vi "Image Processing with Vision Assistant (FPGA)-useFIFO1out.vi"() -> ()   [LabVIEW 2016]
uses:
  <vilib>/visionFPGA/Controls/IMAQ FPGA Image Size.ctl
  <vilib>/rvi/Emulation/niFpgaSctlEmulationGetInTimedLoop.vi
  <vilib>/rvi/Emulation/niFpgaProcessEmulError.vi
  <vilib>/rvi/Emulation/niFpgaGetClockAttributes.vi
  <vilib>/rvi/Emulation/niFpgaEmulationReportErrorSimple.vi
  <vilib>/rvi/eio/common/nirviEmuTemplateMethod_errors.vi
  <vilib>/rvi/interface/RandomDataEmulation/niFpgaRandomDataHandleErrors.vi
  <vilib>/rvi/DataTransferAndStorage/Container/Common/niFpgaContainerGetUniqueNameForEmu.vi
  <vilib>/rvi/DataTransferAndStorage/Container/Common/niFpgaContainerSetEmuInfo.vi
  <vilib>/rvi/eio/common/nirviEmuReportErrorAndStop.vi
  <vilib>/rvi/DataTransferAndStorage/Container/Common/niFpgaContainerExecOnDevCompGetState.vi
  <vilib>/rvi/Emulation/niFpgaEmulationIsFPGAContextNoSignature.vi
  <vilib>/rvi/errors/niFpgaSetErrorForExecOnDevCompSimple.vi
  <vilib>/rvi/FIFO/Fifo_Resource/nirvififoEmulationSetSize.vi
  <vilib>/rvi/FIFO/Fifo_Resource/nirviFifoEmulationQueueMgr.vi
  <instcachedir>/0/nirviFifoEmulationQueueMgr_E5CAEC123FF24DC58D834DCA3CDAA9B5.lvgen/nirviFifoEmulationQueueMgr_E5CAEC123FF24DC58D834DCA3CDAA9B5_002.vi
  <vilib>/rvi/FIFO/Fifo_Resource/nirvififoEmulationDetermineInputValidOut.vi
  <vilib>/rvi/FIFO/Fifo_Resource/nirvififoEmulationCreateLock.vi
  <vilib>/rvi/FIFO/Fifo_Resource/nirvififoEmulationObtainLock.vi
  <vilib>/rvi/FIFO/Fifo_Resource/nirvififoEmulationReleaseLock.vi
  <vilib>/rvi/occurrence/nirviWaitOnOccurrenceBase.vi
  <vilib>/rvi/errors/nirviReportUnexpectedCaseInternalError.vi
  <vilib>/rvi/errors/nirviReportUnexpectedCaseInternalError (U32).vi
  <vilib>/Utility/error.llb/Clear Errors.vi
  <vilib>/rvi/Emulation/niFpgaCriticalErrorInLSC.vi
  <vilib>/eio/EIONode/EIONode.xnode
  <vilib>/rvi/DataTransferAndStorage/Container/XNode/niFpgaContainer.xnode
  <vilib>/rvi/interface/RandomDataEmulation/nirviRandomDataFpgaReadWriteTemplate.vi
  <vilib>/rvi/LocalResourceManager/LocalResourceManager.xnode
  <vilib>/rvi/FIFO/Fifo_Resource/niFpgaFifoEmulationRefIn.vi
panel:
  out "OutputType":u8
  out "CanSendImage":bool=TRUE
  out "Mode LED Status":bool=TRUE
  out "Radio LED Status":bool=TRUE
  out "outputExtreme2":bool=TRUE
  out "outputExtreme1":bool=TRUE
  out "outputDOG2":bool=TRUE
  out "outputDOG1":bool=TRUE
  out "Ready For Output":bool=TRUE
  out "StartOfImage":bool=TRUE
  in  "Image Size":T1={"Width"=640, "Height"=480}
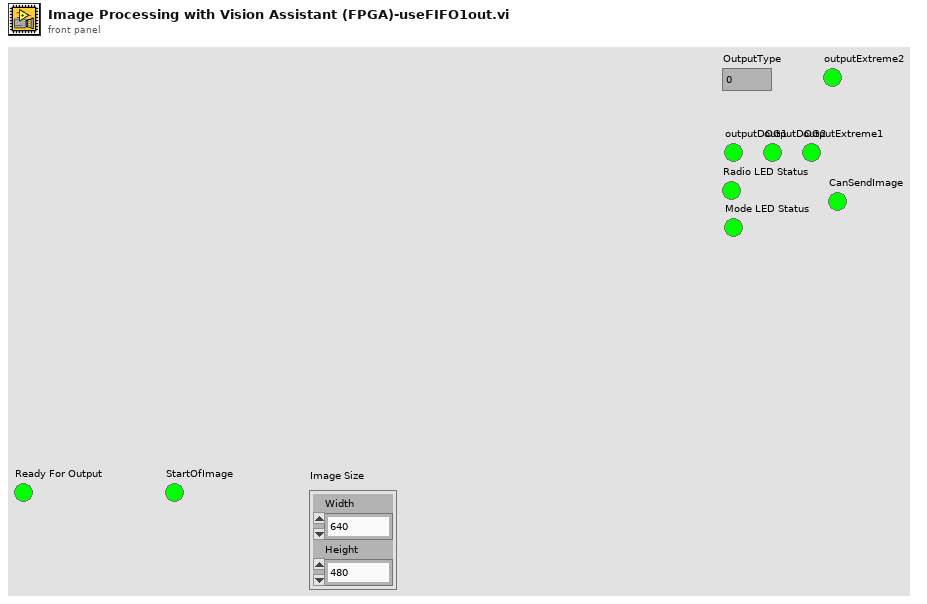
[diagram p1: front panel]
types:
  T1 = typedef "IMAQ FPGA Image Size.ctl" = cluster{"Width":u32, "Height":u32}
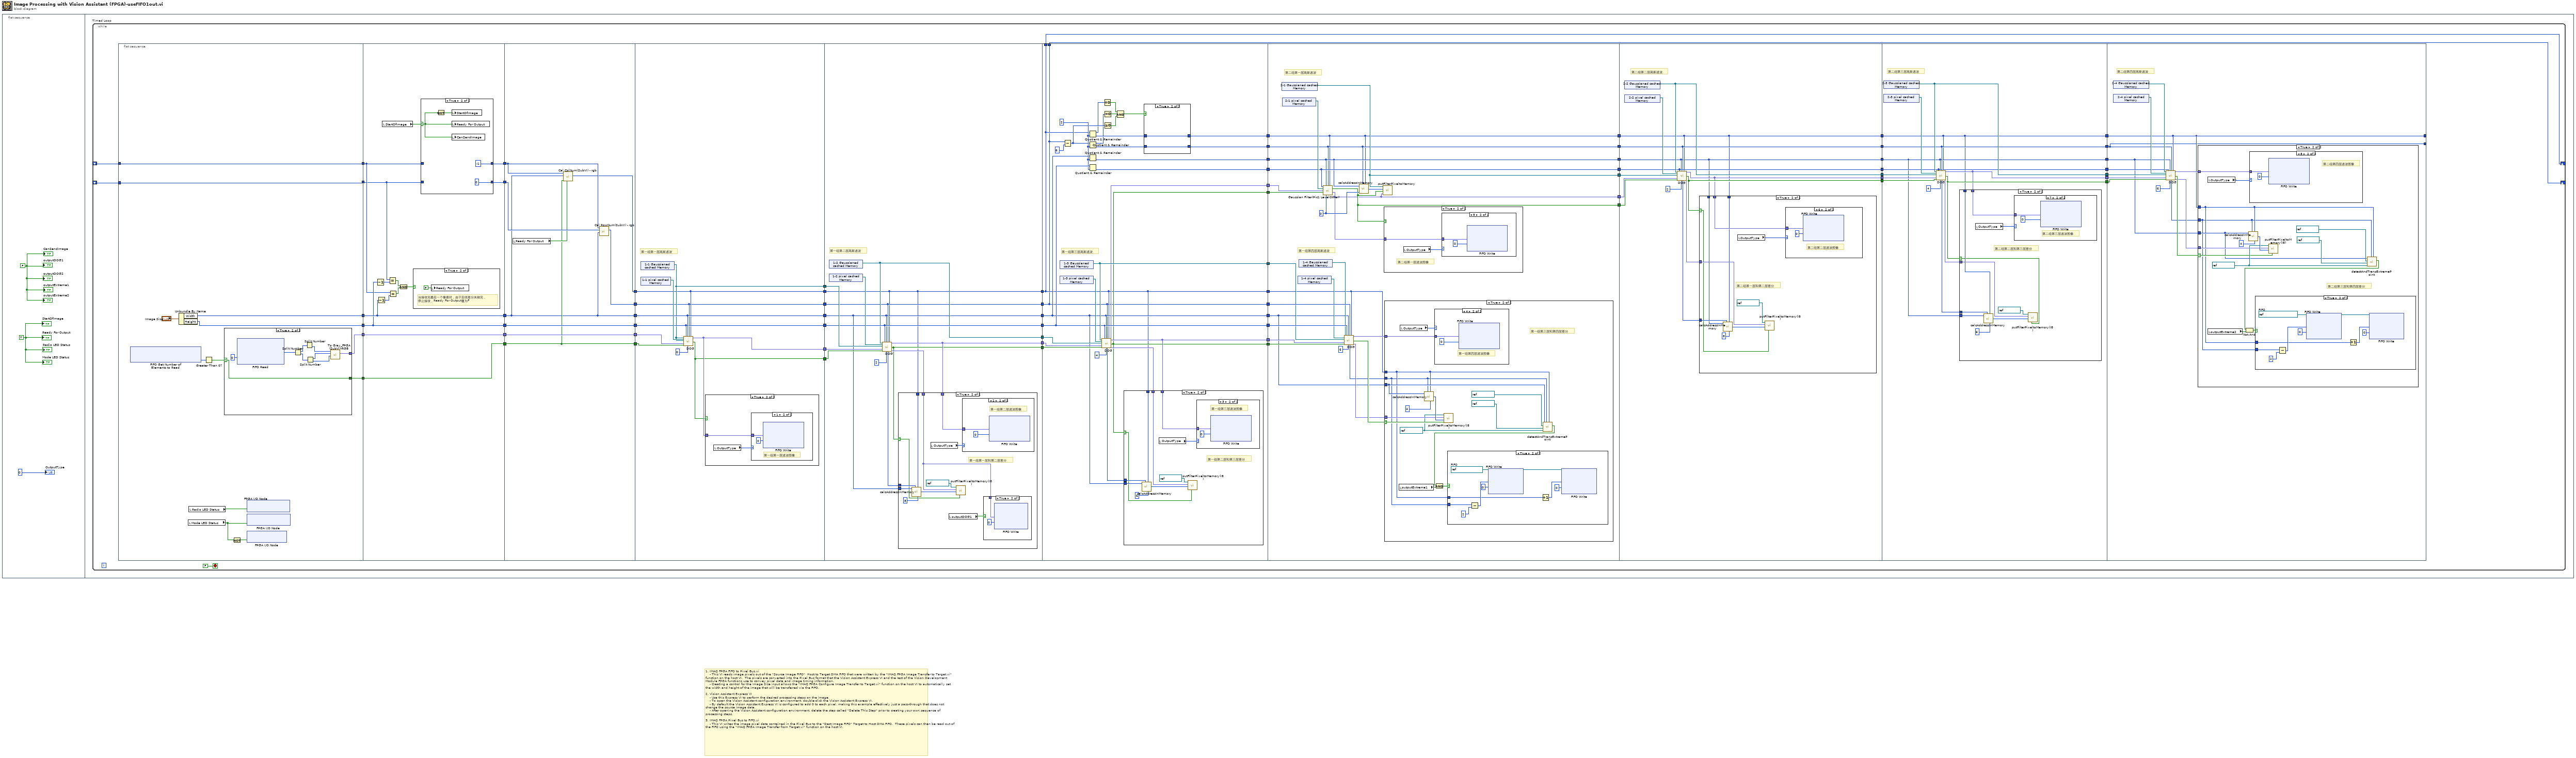
[diagram p0: block diagram]
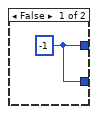
[diagram p10: hidden frame]
diagram:
  # "1. IMAQ FPGA FIFO to Pixel Bus.vi\n    - This VI reads image pixels out of the \"Source Image FIFO\"  Host to Target DMA FIFO that were written by the \"IMAQ FPGA Image Transfer to Target.vi\" function on the host VI.  The pixels are converted into the Pixel Bus format that the Vision Assistant Express VI and the rest of the Vision Development Module FPGA functions use to convey pixel data and image timing information.\n    - Creating a control for the Image Size input allows the \"IMAQ FPGA Configure Image Transfer to Target.vi\" function on the host VI to automatically set the width and height of the image that will be transferred via the FIFO.\n\n2. Vision Assistant Express VI\n    - Use this Express VI to perform the desired processing steps on the image.\n    - To open the Vision Assistant configuration environment, double-click the Vision Assistant Express VI.\n    - By default the Vision Assistant Express VI is configured to add 0 to each pixel, making this example effectively just a pass-through that does not change the source image data.\n    - After opening the Vision Assistant configuration environment, delete the step called \"Delete This Step\" prior to creating your own sequence of processing steps.\n\n3. IMAQ FPGA Pixel Bus to FIFO.vi\n    - This VI writes the image pixel data contained in the Pixel Bus to the \"Dest Image FIFO\" Target to Host DMA FIFO.  These pixels can then be read out of the FIFO using the \"IMAQ FPGA Image Transfer from Target.vi\" function on the host VI."
  n1 = flat-sequence {
    frame #0 {
      w1 = FALSE
      w3 = TRUE ("Ready For Output")
      "StartOfImage" <- w3
      "Ready For Output" <- w3
      "outputDOG1" <- w1
      "outputDOG2" <- w1
      "outputExtreme1" <- w1
      "outputExtreme2" <- w1
      "Radio LED Status" <- w3
      "Mode LED Status" <- w3
      "CanSendImage" <- w1
      "OutputType" <- i16 0
    }
    frame #1 {
      n2 = while "Timed Loop" {
        shift-right: [w10] -> _
        shift-left: _ -> [w14]
        shift-right: [w11] -> _
        shift-left: _ -> [w16]
        stop <- FALSE stop-if-true
        n3 = flat-sequence {
          tunnel: [w85] -> w21
          tunnel: [w84] -> w20
          tunnel: [w78] -> w19
          tunnel: [w77] -> w18
          tunnel: [w76] -> w17
          tunnel: w16 -> [w76]
          tunnel: [w75] -> w15
          tunnel: w14 -> [w75]
          tunnel: [w105] -> w26
          tunnel: [w103] -> w25
          tunnel: [w102] -> w24
          tunnel: [w104] -> w23
          tunnel: w21 -> [w103]
          tunnel: w20 -> [w102]
          tunnel: w19 -> [w105]
          tunnel: w18 -> [w104]
          tunnel: w17 -> [w100]
          tunnel: w15 -> [w99]
          tunnel: [w98] -> w13
          tunnel: [w97] -> w12
          tunnel: [w119] -> w4
          tunnel: [w126] -> w8
          tunnel: [w120] -> w6
          tunnel: [w125] -> w7
          tunnel: [w121] -> w9
          tunnel: w26 -> [w126]
          tunnel: w25 -> [w120]
          tunnel: w24 -> [w125]
          tunnel: w23 -> [w121]
          tunnel: w13 -> [w123]
          tunnel: w12 -> [w124]
          tunnel: [w118] -> w5
          tunnel: w9 -> [w127]
          tunnel: w8 -> [w137]
          tunnel: w7 -> [w133]
          tunnel: w6 -> [w134]
          tunnel: w5 -> [w129]
          tunnel: w4 -> [w128]
          tunnel: [w129] -> w74
          tunnel: [w128] -> w73
          tunnel: [w134] -> w72
          tunnel: [w133] -> w71
          tunnel: [w136] -> w70
          tunnel: [w130] -> w69
          tunnel: [w131] -> w66
          tunnel: w74 -> [w142]
          tunnel: w73 -> [w148]
          tunnel: w72 -> [w144]
          tunnel: w71 -> [w150]
          tunnel: w70 -> [w152]
          tunnel: w69 -> [w151]
          tunnel: [w145] -> w68
          tunnel: [w147] -> w67
          tunnel: w66 -> [w153]
          tunnel: [w142] -> w65
          tunnel: [w148] -> w64
          tunnel: [w144] -> w63
          tunnel: [w150] -> w62
          tunnel: [w149] -> w54
          tunnel: w68 -> [w199]
          tunnel: w67 -> [w198]
          tunnel: w65 -> [w172]
          tunnel: w64 -> [w171]
          tunnel: w63 -> [w173]
          tunnel: w62 -> [w191]
          tunnel: [w177] -> w61
          tunnel: [w175] -> w60
          tunnel: [w172] -> w59
          tunnel: [w171] -> w58
          tunnel: [w173] -> w57
          tunnel: [w191] -> w56
          tunnel: [w196] -> w55
          tunnel: w54 -> [w195]
          tunnel: [w192] -> w53
          tunnel: [w189] -> w52
          tunnel: [w183] -> w51
          tunnel: [w184] -> w50
          tunnel: [w177] -> w49
          tunnel: [w175] -> w48
          tunnel: [w172] -> w11
          tunnel: [w171] -> w10
          tunnel: w61 -> [w240]
          tunnel: w60 -> [w239]
          tunnel: w59 -> [w215]
          tunnel: w58 -> [w238]
          tunnel: w57 -> [w217]
          tunnel: w56 -> [w237]
          tunnel: w55 -> [w234]
          tunnel: w53 -> [w225]
          tunnel: w52 -> [w226]
          tunnel: w51 -> [w224]
          tunnel: w50 -> [w223]
          tunnel: w49 -> [w228]
          tunnel: w48 -> [w229]
          tunnel: [w231] -> w47
          tunnel: [w220] -> w46
          tunnel: [w221] -> w45
          tunnel: [w226] -> w44
          tunnel: [w225] -> w43
          tunnel: [w224] -> w42
          tunnel: [w223] -> w41
          tunnel: w47 -> [w282]
          tunnel: w46 -> [w281]
          tunnel: w45 -> [w280]
          tunnel: w44 -> [w278]
          tunnel: w43 -> [w271]
          tunnel: w42 -> [w277]
          tunnel: w41 -> [w273]
          tunnel: [w279] -> w40
          tunnel: [w273] -> w39
          tunnel: [w277] -> w38
          tunnel: [w271] -> w37
          tunnel: [w278] -> w36
          tunnel: [w274] -> w35
          tunnel: [w276] -> w34
          tunnel: w40 -> [w308]
          tunnel: w39 -> [w297]
          tunnel: w38 -> [w304]
          tunnel: w37 -> [w299]
          tunnel: w36 -> [w303]
          tunnel: w35 -> [w307]
          tunnel: w34 -> [w306]
          tunnel: [w301] -> w33
          tunnel: [w302] -> w32
          tunnel: [w305] -> w31
          tunnel: [w297] -> w30
          tunnel: [w304] -> w29
          tunnel: [w299] -> w28
          tunnel: [w303] -> w27
          tunnel: w33 -> [w333]
          tunnel: w32 -> [w332]
          tunnel: w31 -> [w331]
          tunnel: w30 -> [w324]
          tunnel: w29 -> [w323]
          tunnel: w28 -> [w326]
          tunnel: w27 -> [w330]
          tunnel: [w324] -> _
          tunnel: [w323] -> _
          frame #0 {
            n4 = xnode "FIFO Get Number of Elements to Read"() -> ("Number of Elements to Read"=w80:u32)  [unwired: 1 in, 1 out]
            n5 = Unbundle By Name("Image Size") -> ("Width"=w85:u32, "Height"=w84:u32)
            n6 = local read "Mode LED Status"() -> (w83:bool)
            n7 = local read "Radio LED Status"() -> (w81:bool)
            n8 = Greater Than 0?(x=w80) -> (x > 0?=w79:bool)
            n9 = case shown="True" w79 {
              selector: w79 -> [w87 w88]
              tunnel: [_ w89] -> w78
              tunnel: [w87 w88] -> w77
              frame False {
              }
              frame True {
                n10 = xnode "FIFO Read"("Timeout"=0) -> ("Element"=w96:u32)  [unwired: 1 in, 2 out]
                n11 = Split Number(x=w96) -> (hi(x)=w94:u16, lo(x)=w95:u16)
                n12 = Split Number(x=w94) -> (lo(x)=w93:u8)  [unwired: 1 out]
                n13 = Split Number(x=w95) -> (hi(x)=w92:u8, lo(x)=w91:u8)
                n14 = call "To Gray_FPGA (SubVI)-RGB.vi"("B"=w91, "G"=w92, "R"=w93) -> ("Data Out"=w89:fxp<+,8,8>)  [unwired: 8 in]
              }
            }
            n15 = Not(x=w83) -> (.not. x?=w82:bool)
            n16 = xnode "FPGA I/O Node"("Radio LED Green"=w81) -> ()  [unwired: 1 in, 1 out]
            n17 = xnode "FPGA I/O Node"("Mode LED Green"=w83) -> ()  [unwired: 1 in, 1 out]
            n18 = xnode "FPGA I/O Node"("Mode LED Red"=w82) -> ()  [unwired: 1 in, 1 out]
          }
          frame #1 {
            n19 = Decrement(x=w102) -> (x-1=w108:u32)
            n20 = Decrement(x=w103) -> (x-1=w107:u32)
            n21 = local read "StartOfImage"() -> (w101:bool)
            n22 = Equal?(x=w99, y=w108) -> (x = y?=w110:bool)
            n23 = Equal?(x=w100, y=w107) -> (x = y?=w109:bool)
            n24 = And(x=w110, y=w109) -> (x .and. y?=w106:bool)
            n25 = case shown="True" w106 {
              frame False {
              }
              frame True {
                # "当接收完最后一个像素时，由于后续差分未做完，\n停止接收，Ready For Output置为F"
                n26 = local write "Ready For Output"(FALSE ("Ready For Output")) -> ()
              }
            }
            n27 = case shown="True" w101 {
              selector: w101 -> [_ w113]
              tunnel: w100 -> [w112 _]
              tunnel: w99 -> [w111 _]
              tunnel: [w112 i16 -1] -> w98
              tunnel: [w111 i16 0] -> w97
              frame False {
              }
              frame True {
                n28 = Not(x=w113) -> (.not. x?=w114:bool)
                n29 = local write "StartOfImage"(w114) -> ()
                n30 = local write "Ready For Output"(w113) -> ()
                n31 = local write "CanSendImage"(w113) -> ()
              }
            }
          }
          frame #2 {
            n32 = local read "Ready For Output"() -> (w122:bool)
            n33 = call "Cal ColNum(SubVI) - rgb.vi"("Ready For Input"=w122, "DV"=w121, "Width"=w120, "preCol"=w123) -> ("curCol"=w118:u16)  [unwired: 7 in]
            n34 = call "Cal RowNum(SubVI) - rgb.vi"("Width"=w120, "preRow"=w124, "preCol"=w123) -> ("curRow"=w119:u16)  [unwired: 8 in]
          }
          frame #3 {
            # "第一组第一层高斯滤波"
            n35 = xnode "1-1 Gaussianed cached Memory"() -> ("Memory Out"=w131:refnum<k21>)
            n36 = xnode "1-1 pixel cached Memory"() -> ("Memory Out"=w135:refnum<k21>)
            n37 = call "DOG.vi"("Gaussianed cached Memory"=w131, "pixel cached Memory"=w135, "preGaussianed cached Memory"=w131, "Data in"=w137, "DV in"=w127, "Height"=w133, "Width"=w134, "DelayRowCount"=i16 0, "Rows"=w128, "Cols"=w129) -> ("GaussianFilterData out"=w136:fxp<+,12,12>, "DV out"=w130:bool)  [unwired: 6 in, 2 out]
            n38 = case shown="True" w130 {
              tunnel: w136 -> [_ w139]
              frame False {
              }
              frame True {
                n39 = local read "OutputType"() -> (w138:u8)
                n40 = case shown="1" w138 {
                  tunnel: w139 -> [_ w140]
                  frame 0, Default {
                  }
                  frame 1 {
                    # "第一组第一层滤波图像"
                    n41 = xnode ("FIFO Write")("Element"=w140, "Timeout"=0) -> ()  [unwired: 1 in, 2 out]
                  }
                }
              }
            }
          }
          frame #4 {
            # "第一组第二层高斯滤波"
            n42 = xnode "1-2 Gaussianed cached Memory"() -> ("Memory Out"=w149:refnum<k21>)
            n43 = xnode "1-2 pixel cached Memory"() -> ("Memory Out"=w154:refnum<k21>)
            n44 = call "DOG.vi"("Gaussianed cached Memory"=w149, "pixel cached Memory"=w154, "preGaussianed cached Memory"=w153, "Data in"=w152, "DV in"=w151, "Height"=w150, "Width"=w144, "DelayRowCount"=i16 2, "Rows"=w148, "Cols"=w142) -> ("out Row"=w143:u16, "GaussianFilterData out"=w147:fxp<+,12,12>, "DV out"=w145:bool, "DOG Out"=w146:fxp<+/-,13,13>)  [unwired: 6 in]
            n45 = case shown="True" w145 {
              selector: w145 -> [_ w159]
              tunnel: w147 -> [_ w166]
              tunnel: w146 -> [_ w157]
              tunnel: w144 -> [_ w165]
              tunnel: w143 -> [_ w164]
              tunnel: w142 -> [_ w163]
              frame False {
              }
              frame True {
                # "第一组第一层和第二层差分"
                n46 = call "calcAddressInMemory.vi"("Width"=w165, "Rows"=w164, "Cols"=w163, "divider"=u8 8) -> ("addressInMemory"=w161:u16)  [unwired: 5 in]
                n47 = local read "OutputType"() -> (w158:u8)
                n48 = local read "outputDOG1"() -> (w156:bool)
                n49 = call "putFilterPixeltoMemory(I8).vi"("DV in"=w159, "addressInMemory"=w161, "Data In"=w157, "Memory in"=refnum<k21> "DOG1-1") -> ()  [unwired: 8 in]
                n50 = case shown="2" w158 {
                  tunnel: w166 -> [_ w169]
                  frame 0, Default {
                  }
                  frame 2 {
                    # "第一组第二层滤波图像"
                    n51 = xnode ("FIFO Write")("Element"=w169, "Timeout"=0) -> ()  [unwired: 1 in, 2 out]
                  }
                }
                n52 = case shown="True" w156 {
                  tunnel: w157 -> [_ w168]
                  frame False {
                  }
                  frame True {
                    n53 = xnode "FIFO Write"("Element"=w168, "Timeout"=0) -> ()  [unwired: 1 in, 2 out]
                  }
                }
              }
            }
          }
          frame #5 {
            w190 = u32 2 ("y")
            # "第一组第三层高斯滤波"
            n54 = xnode "1-3 pixel cached Memory"() -> ("Memory Out"=w197:refnum<k21>)
            n55 = xnode "1-3 Gaussianed cached Memory"() -> ("Memory Out"=w196:refnum<k21>)
            n56 = Subtract(x=w171, y=i16 6) -> (x-y=w180:u16)
            n57 = Quotient & Remainder(x=w172, y=w190) -> (x-y*floor(x/y)=w179:u32, floor(x/y)=w181:u32)
            n58 = Quotient & Remainder(x=w180, y=w190) -> (x-y*floor(x/y)=w178:u32, floor(x/y)=w182:u32)
            n59 = Quotient & Remainder(x=w173, y=w190) -> (floor(x/y)=w192:u32)  [unwired: 1 out]
            n60 = Quotient & Remainder(x=w191, y=w190) -> (floor(x/y)=w189:u32)  [unwired: 1 out]
            n61 = call "DOG.vi"("Gaussianed cached Memory"=w196, "pixel cached Memory"=w197, "preGaussianed cached Memory"=w195, "Data in"=w198, "DV in"=w199, "Height"=w191, "Width"=w173, "DelayRowCount"=i16 4, "Rows"=w171, "Cols"=w172) -> ("out Row"=w174:u16, "GaussianFilterData out"=w177:fxp<+,12,12>, "DV out"=w175:bool, "DOG Out"=w176:fxp<+/-,13,13>)  [unwired: 6 in]
            n62 = Equal To 0?(x=w179) -> (x = 0?=w188:bool)
            n63 = Equal To 0?(x=w178) -> (x = 0?=w187:bool)
            n64 = Greater Or Equal To 0?(x=w180) -> (x >= 0?=w186:bool)
            n65 = Compound Arithmetic op=AND(w188, w187, w186) -> (w185:bool)
            n66 = case shown="True" w175 {
              selector: w175 -> [_ w204]
              tunnel: w177 -> [_ w212]
              tunnel: w176 -> [_ w205]
              tunnel: w174 -> [_ w208]
              tunnel: w173 -> [_ w207]
              tunnel: w172 -> [_ w206]
              frame False {
              }
              frame True {
                # "第一组第二层和第三层差分"
                n67 = call "calcAddressInMemory.vi"("Width"=w207, "Rows"=w208, "Cols"=w206, "divider"=u8 6) -> ("addressInMemory"=w210:u16)  [unwired: 5 in]
                n68 = local read "OutputType"() -> (w203:u8)
                n69 = call "putFilterPixeltoMemory(I8).vi"("DV in"=w204, "addressInMemory"=w210, "Data In"=w205, "Memory in"=refnum<k21> "DOG1-2") -> ()  [unwired: 8 in]
                n70 = case shown="3" w203 {
                  tunnel: w212 -> [_ w213]
                  frame 0, Default {
                  }
                  frame 3 {
                    # "第一组第三层滤波图像"
                    n71 = xnode ("FIFO Write")("Element"=w213, "Timeout"=0) -> ()  [unwired: 1 in, 2 out]
                  }
                }
              }
            }
            n72 = case shown="True" w185 {
              tunnel: [w200 w202] -> w184
              tunnel: w181 -> [_ w202]
              tunnel: [w200 w201] -> w183
              tunnel: w182 -> [_ w201]
              frame False {
                w200 = i16 -1 ("t")
              }
              frame True {
              }
            }
          }
          frame #6 {
            w222 = i16 0 ("delayRowCount")
            # "第二组第一层高斯滤波"
            # "第一组第四层高斯滤波"
            n73 = xnode "2-1 Gaussianed cached Memory"() -> ("Memory Out"=w231:refnum<k21>)
            n74 = xnode "2-1 pixel cached Memory"() -> ("Memory Out"=w227:refnum<k21>)
            n75 = xnode "1-4 pixel cached Memory"() -> ("Memory Out"=w235:refnum<k21>)
            n76 = xnode "1-4 Gaussianed cached Memory"() -> ("Memory Out"=w236:refnum<k21>)
            n77 = call "Gaussian Filter(Pic1 LevelOther).vi"("Height"=w226, "Width"=w225, "Rows"=w224, "Cols"=w223, "Memory in"=w227, "Data in"=w228, "DV in"=w229, "DelayRowCount"=w222) -> ("DV out"=w221:bool, "Data Out"=w220:fxp<+,8,8>)  [unwired: 5 in, 1 out]
            n78 = call "DOG.vi"("Gaussianed cached Memory"=w236, "pixel cached Memory"=w235, "preGaussianed cached Memory"=w234, "Data in"=w240, "DV in"=w239, "Height"=w237, "Width"=w217, "DelayRowCount"=i16 6, "Rows"=w238, "Cols"=w215) -> ("out Row"=w216:u16, "GaussianFilterData out"=w230:fxp<+,12,12>, "DV out"=w219:bool, "DOG Out"=w218:fxp<+/-,13,13>)  [unwired: 6 in]
            n79 = call "calcAddressInMemory.vi"("Width"=w225, "Rows"=w224, "delayRowCount"=w222, "Cols"=w223) -> ("addressInMemory"=w232:u16)  [unwired: 5 in]
            n80 = call "putFilterPixeltoMemory.vi"("Data In"=w220, "DV in"=w221, "addressInMemory"=w232, "Memory in"=w231) -> ()
            n81 = case shown="True" w221 {
              tunnel: w220 -> [_ w242]
              frame False {
              }
              frame True {
                # "第二组第一层滤波图像"
                n82 = local read "OutputType"() -> (w241:u8)
                n83 = case shown="5" w241 {
                  tunnel: w242 -> [_ w243]
                  frame 0, Default {
                  }
                  frame 5 {
                    n84 = xnode ("FIFO Write")("Element"=w243, "Timeout"=0) -> ()  [unwired: 1 in, 2 out]
                  }
                }
              }
            }
            n85 = case shown="True" w219 {
              selector: w219 -> [_ w255]
              tunnel: w230 -> [_ w259]
              tunnel: w218 -> [_ w256]
              tunnel: w217 -> [_ w254]
              tunnel: w216 -> [_ w248]
              tunnel: w215 -> [_ w249]
              frame False {
              }
              frame True {
                w251 = refnum<k21> "DOG1-3" ("Memory in")
                # "第一组第三层和第四层差分"
                n86 = local read "outputExtreme1"() -> (w246:bool)
                n87 = local read "OutputType"() -> (w250:u8)
                n88 = call "calcAddressInMemory.vi"("Width"=w254, "Rows"=w248, "Cols"=w249, "divider"=u8 4) -> ("addressInMemory"=w257:u16)  [unwired: 5 in]
                n89 = case shown="4" w250 {
                  tunnel: w259 -> [_ w270]
                  frame 0, Default {
                  }
                  frame 4 {
                    # "第一组第四层滤波图像"
                    n90 = xnode ("FIFO Write")("Element"=w270, "Timeout"=0) -> ()  [unwired: 1 in, 2 out]
                  }
                }
                n91 = call "putFilterPixeltoMemory(I8).vi"("DV in"=w255, "addressInMemory"=w257, "Data In"=w256, "Memory in"=w251) -> ()  [unwired: 8 in]
                n92 = call "detectAndTransExtremePoint.vi"("Col"=w249, "Row"=w248, "Level3 Memory"=w251, "Level2 Memory"=refnum<k21> "DOG1-2" ("Memory In"), "Level1 Memory"=refnum<k21> "DOG1-1" ("Memory In"), "Width"=w254) -> ("isExtreme?"=w245:bool)  [unwired: 5 in]
                n93 = And(x=w245, y=w246) -> (x .and. y?=w247:bool)
                n94 = case shown="True" w247 {
                  tunnel: w248 -> [_ w267]
                  tunnel: w249 -> [_ w261]
                  frame False {
                  }
                  frame True {
                    w260 = refnum<k21> "extreme FIFO"  # FIFO
                    n95 = Subtract(x=w267, y=u16 2) -> (x-y=w265:u16)
                    n96 = xnode ("FIFO Write")("Element"=w265, "Timeout"=0, "FIFO In"=w260) -> ("FIFO Out"=w263:refnum<k21>)  [unwired: 1 out]
                    n97 = Increment(x=w261) -> (x+1=w262:u16)
                    n98 = xnode ("FIFO Write")("Element"=w262, "Timeout"=0, "FIFO In"=w263) -> ()  [unwired: 2 out]
                  }
                }
              }
            }
          }
          frame #7 {
            # "第二组第二层高斯滤波"
            n99 = xnode "2-2 Gaussianed cached Memory"() -> ("Memory Out"=w279:refnum<k21>)
            n100 = xnode "2-2 pixel cached Memory"() -> ("Memory Out"=w283:refnum<k21>)
            n101 = call "DOG.vi"("Gaussianed cached Memory"=w279, "pixel cached Memory"=w283, "preGaussianed cached Memory"=w282, "Data in"=w281, "DV in"=w280, "Height"=w278, "Width"=w271, "DelayRowCount"=i16 2, "Rows"=w277, "Cols"=w273) -> ("out Row"=w272:u16, "GaussianFilterData out"=w274:fxp<+,12,12>, "DV out"=w276:bool, "DOG Out"=w275:fxp<+/-,13,13>)  [unwired: 6 in]
            n102 = case shown="True" w276 {
              selector: w276 -> [_ w286]
              tunnel: w275 -> [_ w287]
              tunnel: w274 -> [_ w294]
              tunnel: w273 -> [_ w290]
              tunnel: w272 -> [_ w289]
              tunnel: w271 -> [_ w288]
              frame False {
              }
              frame True {
                # "第二组第一层和第二层差分"
                n103 = call "calcAddressInMemory.vi"("Width"=w288, "Rows"=w289, "Cols"=w290, "divider"=u8 8) -> ("addressInMemory"=w292:u16)  [unwired: 5 in]
                n104 = local read "OutputType"() -> (w285:u8)
                n105 = call "putFilterPixeltoMemory(I8).vi"("DV in"=w286, "addressInMemory"=w292, "Data In"=w287, "Memory in"=refnum<k21> "DOG2-1") -> ()  [unwired: 8 in]
                n106 = case shown="6" w285 {
                  tunnel: w294 -> [_ w295]
                  frame 0, Default {
                  }
                  frame 6 {
                    # "第二组第二层滤波图像"
                    n107 = xnode ("FIFO Write")("Element"=w295, "Timeout"=0) -> ()  [unwired: 1 in, 2 out]
                  }
                }
              }
            }
          }
          frame #8 {
            # "第二组第三层高斯滤波"
            n108 = xnode "2-3 Gaussianed cached Memory"() -> ("Memory Out"=w305:refnum<k21>)
            n109 = xnode "2-3 pixel cached Memory"() -> ("Memory Out"=w309:refnum<k21>)
            n110 = call "DOG.vi"("Gaussianed cached Memory"=w305, "pixel cached Memory"=w309, "preGaussianed cached Memory"=w308, "Data in"=w307, "DV in"=w306, "Height"=w303, "Width"=w299, "DelayRowCount"=i16 4, "Rows"=w304, "Cols"=w297) -> ("out Row"=w298:u16, "GaussianFilterData out"=w301:fxp<+,12,12>, "DV out"=w302:bool, "DOG Out"=w300:fxp<+/-,13,13>)  [unwired: 6 in]
            n111 = case shown="True" w302 {
              selector: w302 -> [_ w312]
              tunnel: w301 -> [_ w320]
              tunnel: w300 -> [_ w313]
              tunnel: w299 -> [_ w316]
              tunnel: w298 -> [_ w315]
              tunnel: w297 -> [_ w314]
              frame False {
              }
              frame True {
                # "第二组第二层和第三层差分"
                n112 = local read "OutputType"() -> (w311:u8)
                n113 = call "calcAddressInMemory.vi"("Width"=w316, "Rows"=w315, "Cols"=w314, "divider"=u8 6) -> ("addressInMemory"=w318:u16)  [unwired: 5 in]
                n114 = case shown="7" w311 {
                  tunnel: w320 -> [_ w322]
                  frame 0, Default {
                  }
                  frame 7 {
                    # "第二组第三层滤波图像"
                    n115 = xnode ("FIFO Write")("Element"=w322, "Timeout"=0) -> ()  [unwired: 1 in, 2 out]
                  }
                }
                n116 = call "putFilterPixeltoMemory(I8).vi"("DV in"=w312, "addressInMemory"=w318, "Data In"=w313, "Memory in"=refnum<k21> "DOG2-2") -> ()  [unwired: 8 in]
              }
            }
          }
          frame #9 {
            # "第二组第四层高斯滤波"
            n117 = xnode "2-4 Gaussianed cached Memory"() -> ("Memory Out"=w334:refnum<k21>)
            n118 = xnode "2-4 pixel cached Memory"() -> ("Memory Out"=w335:refnum<k21>)
            n119 = call "DOG.vi"("Gaussianed cached Memory"=w334, "pixel cached Memory"=w335, "preGaussianed cached Memory"=w331, "Data in"=w333, "DV in"=w332, "Height"=w330, "Width"=w326, "DelayRowCount"=i16 6, "Rows"=w323, "Cols"=w324) -> ("out Row"=w325:u16, "GaussianFilterData out"=w328:fxp<+,12,12>, "DV out"=w329:bool, "DOG Out"=w327:fxp<+/-,13,13>)  [unwired: 6 in]
            n120 = case shown="True" w329 {
              selector: w329 -> [_ w345]
              tunnel: w328 -> [_ w351]
              tunnel: w327 -> [_ w344]
              tunnel: w326 -> [_ w343]
              tunnel: w325 -> [_ w341]
              tunnel: w324 -> [_ w342]
              frame False {
              }
              frame True {
                w346 = refnum<k21> "DOG2-3" ("Memory in")
                # "第二组第三层和第四层差分"
                n121 = local read "OutputType"() -> (w337:u8)
                n122 = local read "outputExtreme2"() -> (w338:bool)
                n123 = call "calcAddressInMemory.vi"("Width"=w343, "Rows"=w341, "Cols"=w342, "divider"=u8 4) -> ("addressInMemory"=w349:u16)  [unwired: 5 in]
                n124 = case shown="8" w337 {
                  tunnel: w351 -> [_ w353]
                  frame 0, Default {
                  }
                  frame 8 {
                    # "第二组第四层滤波图像"
                    n125 = xnode ("FIFO Write")("Element"=w353, "Timeout"=0) -> ()  [unwired: 1 in, 2 out]
                  }
                }
                n126 = call "putFilterPixeltoMemory(I8).vi"("DV in"=w345, "addressInMemory"=w349, "Data In"=w344, "Memory in"=w346) -> ()  [unwired: 8 in]
                n127 = call "detectAndTransExtremePoint.vi"("Col"=w342, "Row"=w341, "Level3 Memory"=w346, "Level2 Memory"=refnum<k21> "DOG2-2" ("Memory In"), "Level1 Memory"=refnum<k21> "DOG2-1" ("Memory In"), "Width"=w343) -> ("isExtreme?"=w339:bool)  [unwired: 5 in]
                n128 = Not And(1:w338, 2:w339) -> (0:w340:bool)
                n129 = case shown="True" w340 {
                  tunnel: w341 -> [_ w361]
                  tunnel: w342 -> [_ w355]
                  frame False {
                  }
                  frame True {
                    w354 = refnum<k21> "extreme FIFO dec"  # FIFO
                    n130 = Subtract(x=w361, y=u16 2) -> (x-y=w359:u16)
                    n131 = xnode ("FIFO Write")("Element"=w359, "Timeout"=0, "FIFO In"=w354) -> ("FIFO Out"=w357:refnum<k21>)  [unwired: 1 out]
                    n132 = Increment(x=w355) -> (x+1=w356:u32)
                    n133 = xnode ("FIFO Write")("Element"=w356, "Timeout"=0, "FIFO In"=w357) -> ()  [unwired: 2 out]
                  }
                }
              }
            }
          }
        }
      }
    }
  }
